vi "Test-ListSharedDependencies.vi"() -> ()   [LabVIEW 2013]
uses:
  SMO/SMO.lvclass
  SMO.SelfTerminatingOverride/SMO.SelfTerminatingOverride.lvclass
panel:
  out "[Dependencies] 2":refnum<class "SMO.lvclass">[](array[class])
  out "[Dependencies]":refnum<class "SMO.lvclass">[](array[class])
  out "error out":errorcluster
  # "<< Should have two dependencies"
  # "<< Should have one dependency"
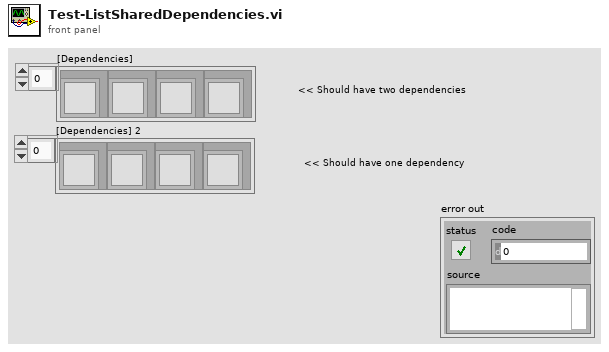
[diagram p1: front panel]
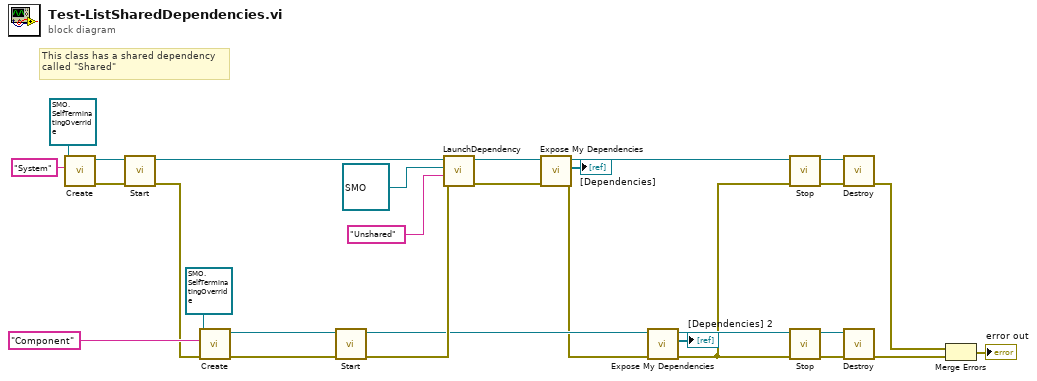
[diagram p0: block diagram]
diagram:
  # "This class has a shared dependency\ncalled \"Shared\""
  n1 = call "Create.vi"("Subsystem Name (optional)"="System", "SMO"=refnum<class "SMO.SelfTerminatingOverride.lvclass"> refnum ("SMO.SelfTerminatingOverride.lvclass")) -> ("error out"=w27:errorcluster, "SMO out"=w28:refnum<class "SMO.SelfTerminatingOverride.lvclass">)  [unwired: 7 in, 1 out]
  n2 = call "Start.vi"("error in (no error)"=w27, "SMO"=w28) -> ("error out"=w20:errorcluster, "SMO out"=w17:refnum<class "SMO.SelfTerminatingOverride.lvclass">)  [unwired: 8 in]
  n3 = call "Create.vi"("error in (no error)"=w20, "Subsystem Name (optional)"="Component", "SMO"=refnum<class "SMO.SelfTerminatingOverride.lvclass"> refnum ("SMO.SelfTerminatingOverride.lvclass")) -> ("error out"=w19:errorcluster, "SMO out"=w21:refnum<class "SMO.SelfTerminatingOverride.lvclass">)  [unwired: 6 in, 1 out]
  n4 = call "Start.vi"("error in (no error)"=w19, "SMO"=w21) -> ("error out"=w13:errorcluster, "SMO out"=w11:refnum<class "SMO.SelfTerminatingOverride.lvclass">)  [unwired: 8 in]
  n5 = call "LaunchDependency.vi"("error in (no error)"=w13, "Dependency Name"="Unshared" ("Subsystem Name (optional)"), "Dependency Type"=refnum<class "SMO.lvclass"> refnum, "SMO in"=w17) -> ("error out"=w12:errorcluster, "SMO out"=w16:refnum<class "SMO.SelfTerminatingOverride.lvclass">)  [unwired: 4 in, 2 out]
  n6 = call "Expose My Dependencies.vi"("error in (no error)"=w12, "SMO.SelfTerminatingOverride in"=w16) -> ("error out"=w10:errorcluster, "[Dependencies]"=→"[Dependencies]":refnum<class "SMO.lvclass">[], "SMO.SelfTerminatingOverride out"=w18:refnum<class "SMO.SelfTerminatingOverride.lvclass">)  [unwired: 7 in]
  n7 = call "Expose My Dependencies.vi"("error in (no error)"=w10, "SMO.SelfTerminatingOverride in"=w11) -> ("error out"=w6:errorcluster, "[Dependencies]"=→"[Dependencies] 2":refnum<class "SMO.lvclass">[], "SMO.SelfTerminatingOverride out"=w7:refnum<class "SMO.SelfTerminatingOverride.lvclass">)  [unwired: 7 in]
  n8 = call "Stop.vi"("error in (no error)"=w6, "SMO"=w18) -> ("error out"=w24:errorcluster, "SMO out"=w25:refnum<class "SMO.SelfTerminatingOverride.lvclass">)  [unwired: 8 in]
  n9 = call "Stop.vi"("error in (no error)"=w6, "SMO"=w7) -> ("error out"=w9:errorcluster, "SMO out"=w8:refnum<class "SMO.SelfTerminatingOverride.lvclass">)  [unwired: 8 in]
  n10 = call "Destroy.vi"("error in (no error)"=w24, "SMO"=w25) -> ("error out"=w4:errorcluster)  [unwired: 9 in]
  n11 = call "Destroy.vi"("error in (no error)"=w9, "SMO"=w8) -> ("error out"=w5:errorcluster)  [unwired: 9 in]
  n12 = Merge Errors(w4, w5) -> (→"error out":errorcluster)
